vi "N5700 Wait.vi"(5 "error":errorcluster, 7 "Delay (5 mS)":u32=20, 8 "VISA":refnum<visa-resource-name>) -> (0 "error out":errorcluster, 3 "VISA out":refnum<visa-resource-name>)   [LabVIEW 2020]
doc: "Wait number of milliseconds. If \"Delay\" input not wired, it will wait 20 mSec.\n\nIf \"error\" input is set to error, it will not wait"
panel:
  # "Agilent Technologies  \nSeries N5700A\n  DC Power Supplies"
  # "WAIT\nmilliSeconds"
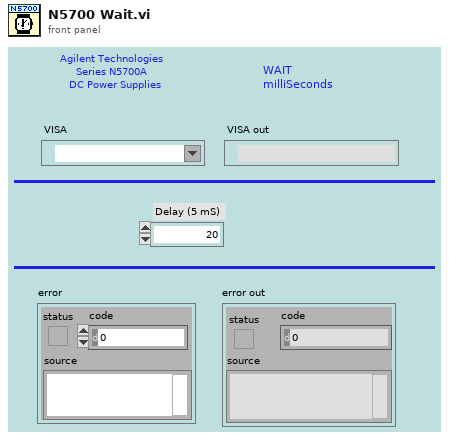
[diagram p1: front panel]
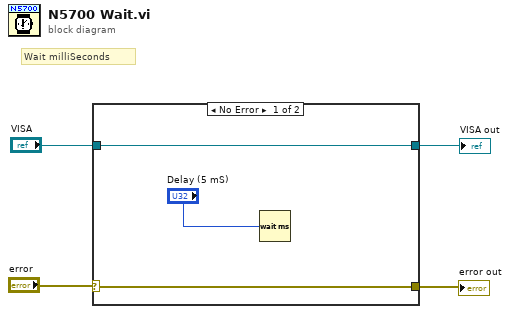
[diagram p0: block diagram]
diagram:
  # "Wait milliSeconds"
  n1 = case shown="No Error" "error" {
    selector: "error" -> [w7 w8]
    tunnel: [w7 w8] -> w3
    tunnel: "VISA" -> [w6 w9]
    tunnel: [w6 w9] -> w1
    frame No Error {
      n2 = Wait (ms)(milliseconds to wait="Delay (5 mS)") -> ()  [unwired: 1 out]
    }
    frame Error {
      # "If Error Exists,  Do Not Wait"
    }
  }
  "error out" <- w3
  "VISA out" <- w1
